vi "UpdateTimesJuicer.vi"(8 "error in (no error)":errorcluster, 9 "Air Duration":dbl format="%#_13g", 10 "Pulse Duration":dbl[](array[numeric]), 11 "Juicer in":refnum<class "Juicer.lvclass">) -> (0 "error out":errorcluster, 2 "Juice":bool[](array[boolean]), 3 "Juicer out":refnum<class "Juicer.lvclass">)   [LabVIEW 2014, in "Juicer.lvclass"]
uses:
  Juicer.lvclass
  Juicer.lvclass/Juicer.ctl
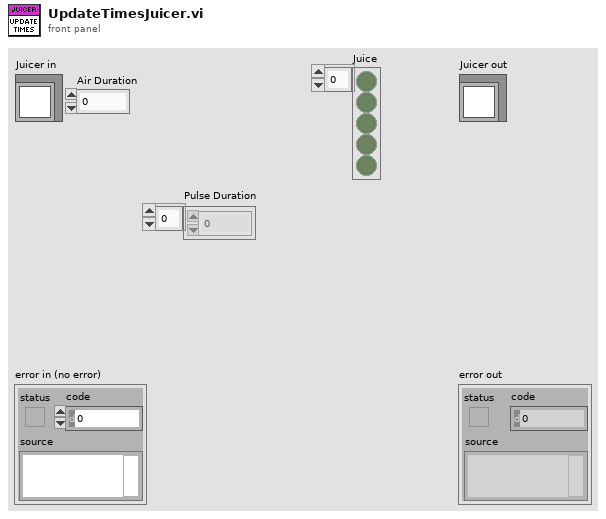
[diagram p1: front panel]
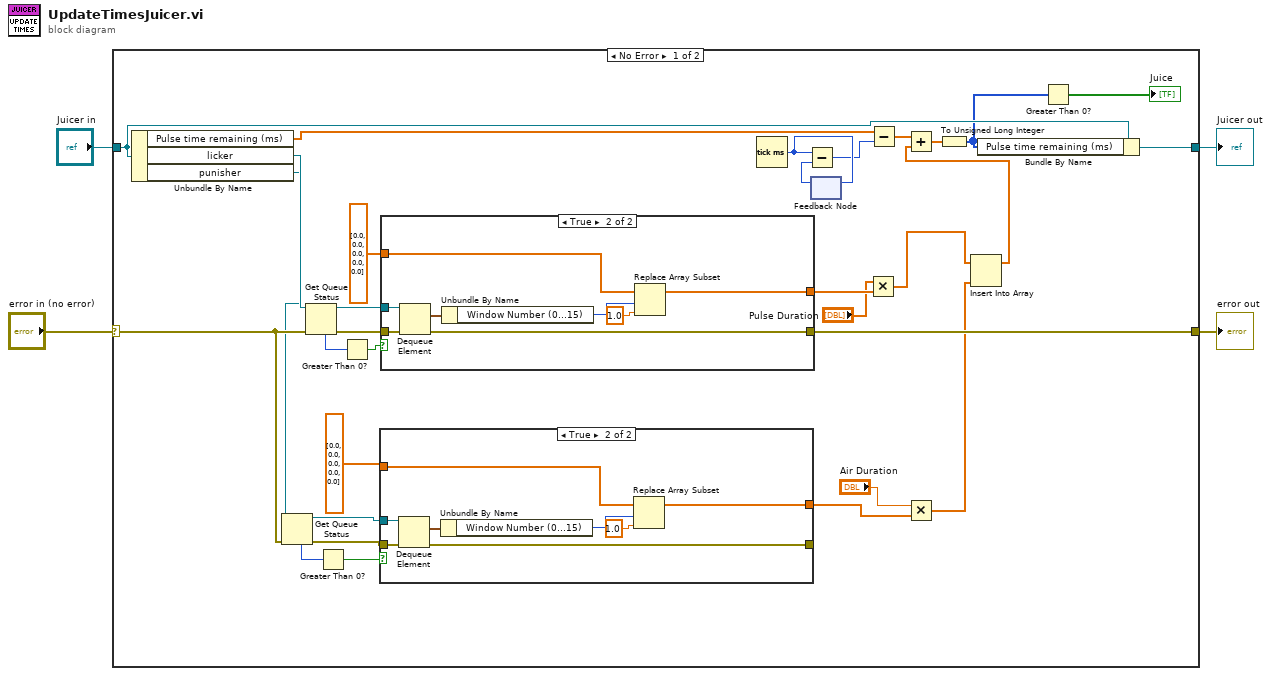
[diagram p0: block diagram]
diagram:
  n1 = case shown="No Error" "error in (no error)" {
    selector: "error in (no error)" -> [w11 w57]
    tunnel: [w26 w57] -> w3
    tunnel: [w28 w56] -> w1
    tunnel: "Juicer in" -> [w29 w56]
    frame No Error {
      n2 = Unbundle By Name(w29) -> ("Pulse time remaining (ms)"=w17:dbl[], "licker"=w22:refnum<queue>, "punisher"=w10:refnum<queue>)
      n3 = Get Queue Status(queue=w10, error in (no error)=w11) -> (queue out=w14:refnum<queue>, error out=w13:errorcluster, # elements in queue=w16:i32)  [unwired: 1 in, 5 out]
      n4 = Get Queue Status(queue=w22, error in (no error)=w11) -> (queue out=w21:refnum<queue>, error out=w20:errorcluster, # elements in queue=w19:i32)  [unwired: 1 in, 5 out]
      n5 = Greater Than 0?(x=w16) -> (x > 0?=w12:bool)
      n6 = Greater Than 0?(x=w19) -> (x > 0?=w18:bool)
      n7 = case shown="True" w12 {
        tunnel: [w37 w45] -> _
        tunnel: dbl[] [0.0, 0.0, 0.0, 0.0, 0.0] -> [w36 w43]
        tunnel: [w36 w40] -> w9
        tunnel: w14 -> [_ w39]
        tunnel: w13 -> [w37 w38]
        frame False {
        }
        frame True {
          n8 = Dequeue Element(queue=w39, error in (no error)=w38) -> (element=w44:cluster{"Window Number (0...15)":i32}, error out=w45:errorcluster)  [unwired: 1 in, 2 out]
          n9 = Unbundle By Name(w44) -> ("Window Number (0...15)"=w42:i32)
          n10 = Replace Array Subset(array=w43, new element=1.0 ("new element/subarray"), index=w42) -> (w40:dbl[])
        }
      }
      n11 = case shown="True" w18 {
        tunnel: [w47 w55] -> w26
        tunnel: dbl[] [0.0, 0.0, 0.0, 0.0, 0.0] -> [w46 w53]
        tunnel: [w46 w50] -> w24
        tunnel: w21 -> [_ w49]
        tunnel: w20 -> [w47 w48]
        frame False {
        }
        frame True {
          n12 = Dequeue Element(queue=w49, error in (no error)=w48) -> (element=w54:cluster{"Window Number (0...15)":i32}, error out=w55:errorcluster)  [unwired: 1 in, 2 out]
          n13 = Unbundle By Name(w54) -> ("Window Number (0...15)"=w52:i32)
          n14 = Replace Array Subset(array=w53, new element=1.0 ("new element/subarray"), index=w52) -> (w50:dbl[])
        }
      }
      n15 = Tick Count (ms)() -> (millisecond timer value=w35:u32)
      n16 = feedback-in #1(w35) -> ()
      n17 = feedback #1() -> (w34:u32)  [unwired: 1 in]
      n18 = Subtract(x=w35, y=w34) -> (x-y=w33:u32)
      n19 = Multiply(x="Pulse Duration", y=w24) -> (x*y=w8:dbl[])
      n20 = Subtract(x=w17, y=w33) -> (x-y=w32:dbl[])
      n21 = Multiply(x="Air Duration", y=w9) -> (x*y=w7:dbl[])
      n22 = Insert Into Array(array=w8, new element=w7) -> (w6:dbl[])  [unwired: 1 in]
      n23 = Add(x=w32, y=w6) -> (x+y=w30:dbl[])
      n24 = To Unsigned Long Integer(number=w30) -> (unsigned 32bit integer=w27:u32[])
      n25 = Bundle By Name(cluster=w29, "Pulse time remaining (ms)"=w27) -> (w28:refnum<class "Juicer.lvclass">)
      n26 = Greater Than 0?(x=w27) -> (x > 0?=→"Juice":bool[])
    }
    frame Error {
    }
  }
  "error out" <- w3
  "Juicer out" <- w1
